vi "Regenerate Energy.vi"(11 "Ship in":refnum<class "Ship.lvclass">) -> (3 "Ship out":refnum<class "Ship.lvclass">)   [LabVIEW 2021, in "Ship.lvclass"]
uses:
  Ship.lvclass
  Ship.lvclass/Ship.ctl
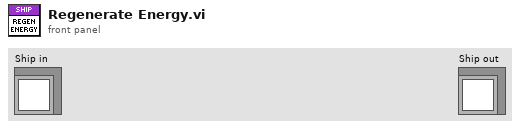
[diagram p1: front panel]
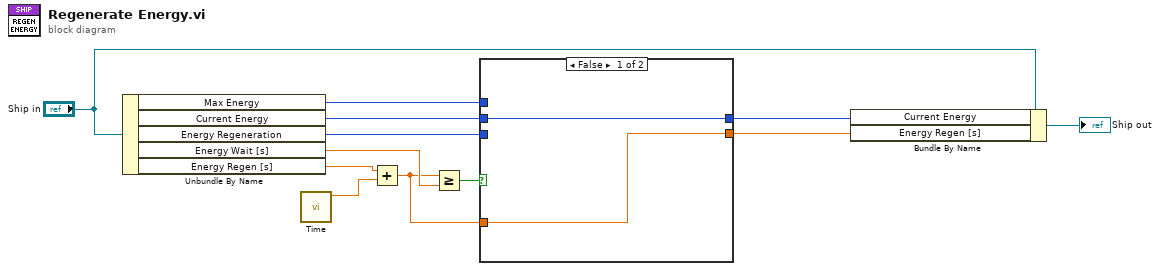
[diagram p0: block diagram]
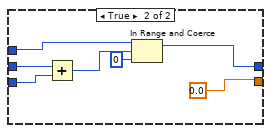
[diagram p2: hidden frame]
diagram:
  n1 = Unbundle By Name("Ship in") -> ("Max Energy"=w1:i32, "Current Energy"=w6:i32, "Energy Regeneration"=w5:i32, "Energy Wait [s]"=w8:sgl, "Energy Regen [s]"=w12:sgl)
  n2 = call "Time.vi"() -> ("Delta Time [s]"=w11:sgl)  [unwired: 10 in, 1 out]
  n3 = Add(x=w12, y=w11) -> (x+y=w3:sgl)
  n4 = Greater Or Equal?(x=w3, y=w8) -> (x >= y?=w7:bool)
  n5 = case shown="False" w7 {
    tunnel: w6 -> [w14 w21]
    tunnel: w5 -> [_ w20]
    tunnel: [w14 w15] -> w4
    tunnel: w3 -> [w13 _]
    tunnel: [w13 0.0] -> w2
    tunnel: w1 -> [_ w18]
    frame False {
    }
    frame True {
      n6 = Add(x=w21, y=w20) -> (x+y=w16:i32)
      n7 = In Range and Coerce(upper limit=w18, x=w16, lower limit=0) -> (coerced(x)=w15:i32)  [unwired: 1 out]
    }
  }
  n8 = Bundle By Name(cluster="Ship in", "Current Energy"=w4, "Energy Regen [s]"=w2) -> (→"Ship out":refnum<class "Ship.lvclass">)
